vi "Spawn.vi"(6 "Start Direction":T1=enum."E", 8 "error in (no error)":errorcluster, 10 "?":T2, 11 "Mother in":refnum<class "Mother.lvclass">) -> (0 "error out":errorcluster, 2 "Replicated Class":refnum<class "Mother.lvclass">, 3 "Mother out":refnum<class "Mother.lvclass">)   [LabVIEW 2014, in "Mother.lvclass"]
uses:
  Mother.lvclass
  Formic Types.ctl
  Direction Enum.ctl
  Mother.lvclass/Mother.ctl
  Scout/Scout.lvclass
  Coward/Coward.lvclass
  Protector/Protector.lvclass
  SquareBattle.lvclass
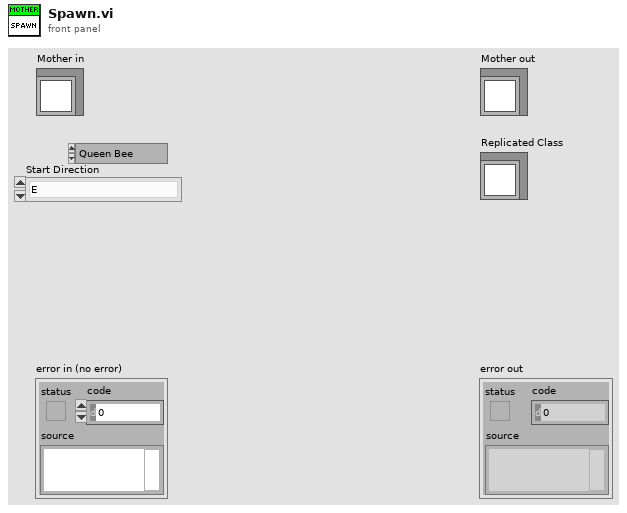
[diagram p1: front panel]
types:
  T1 = typedef "SquareBattle.lvclass/Direction Enum.ctl" = enum16{"NW", "N", "NE", "E", "SE", "S", "SW", "W"}
  T2 = typedef "Mother.lvclass/Formic Types.ctl" = enum16{"Queen Bee", "Protector Bee", "Daughter Bee", "Worker Bee", "Coward"}
  T3 = typedef "Mother.lvclass/SquareStatus DVR.ctl" = refnum<data-value>
  T4 = typedef "Mother.lvclass/Kamikaze DVR.ctl" = refnum<data-value>
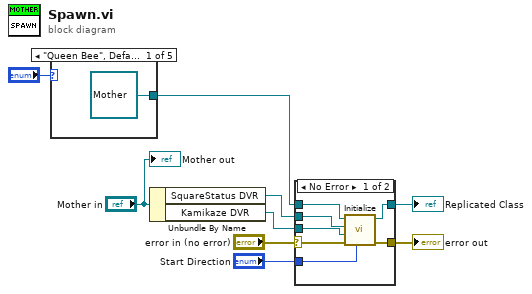
[diagram p0: block diagram]
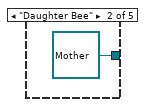
[diagram p2: hidden frame]
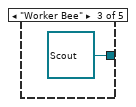
[diagram p3: hidden frame]
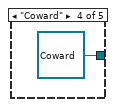
[diagram p4: hidden frame]
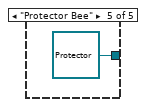
[diagram p5: hidden frame]
diagram:
  n1 = case shown="\"Queen Bee\", Default" "?" {
    tunnel: [refnum<class "Mother.lvclass"> refnum ("Mother.lvclass") refnum<class "Mother.lvclass"> refnum ("Mother.lvclass") refnum<class "Scout.lvclass"> refnum ("Scout.lvclass") refnum<class "Coward.lvclass"> refnum ("Coward.lvclass") refnum<class "Protector.lvclass"> refnum ("Protector.lvclass")] -> w6
    frame "Queen Bee", Default {
    }
    frame "Daughter Bee" {
    }
    frame "Worker Bee" {
    }
    frame "Coward" {
    }
    frame "Protector Bee" {
    }
  }
  n2 = Unbundle By Name("Mother in") -> ("SquareStatus DVR"=w3:T3, "Kamikaze DVR"=w2:T4)
  n3 = case shown="No Error" "error in (no error)" {
    selector: "error in (no error)" -> [w21 w23]
    tunnel: [w20 w23] -> w8
    tunnel: [w18 w22] -> w5
    tunnel: w6 -> [w19 w22]
    tunnel: w3 -> [w17 _]
    tunnel: w2 -> [w16 _]
    tunnel: "Start Direction" -> [w15 _]
    frame No Error {
      n4 = call-dynamic "Initialize.vi"("Start Direction"=w15, "error in (no error)"=w21, "Kamikaze DVR"=w16, "SquareStatus DVR"=w17, "Mother in"=w19) -> ("error out"=w20:errorcluster, "Mother out"=w18:refnum<class "Mother.lvclass">)  [unwired: 5 in]
    }
    frame Error {
    }
  }
  "error out" <- w8
  "Replicated Class" <- w5
  "Mother out" <- "Mother in"
